vi "FRC-Traj-Lib-SlewRateLimiter-Sample-2.vi"() -> ()   [LabVIEW 2019]
uses:
  <vilib>/Rock Robotics/WPI/ThirdParty/JAS_Junk/TrajLib/Trajectory_Library.lvlib
panel:
  in  "Tab Control":enum32{"Control Panel", "Logic"}(tab)
  in  "Rate Limit  \nMax Units/Sec":dbl=10.0
  in  "Raw Input":dbl(slide)=10.0 scale=-100.0..100.0
  out "Rate Limited Output":dbl
  in  "Enable":bool
  out "Trend":cluster{"Input":dbl, "Output":dbl}(graph)
  out "Rate Limiting Enabled":bool
  # "Slew Rate Limiter Sample 2"
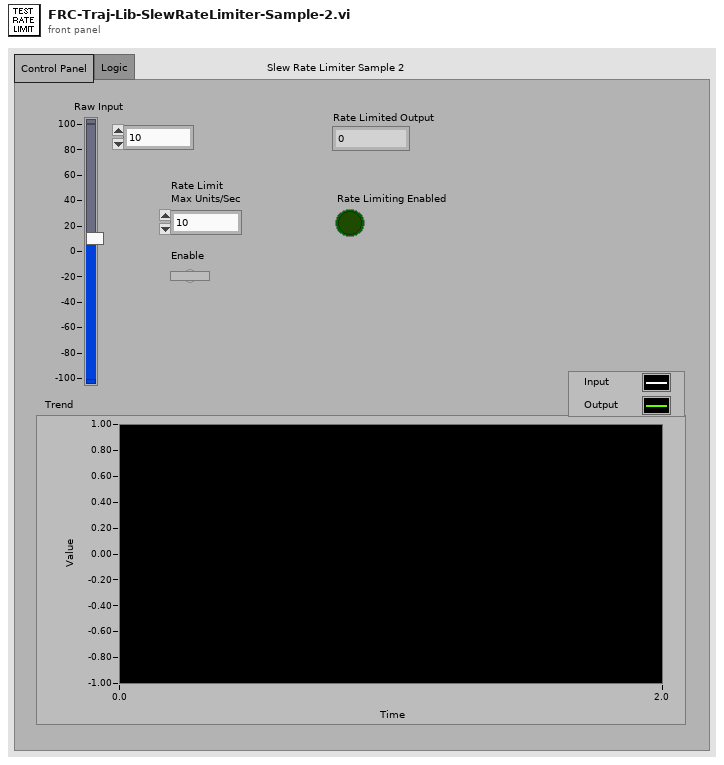
[diagram p1: front panel]
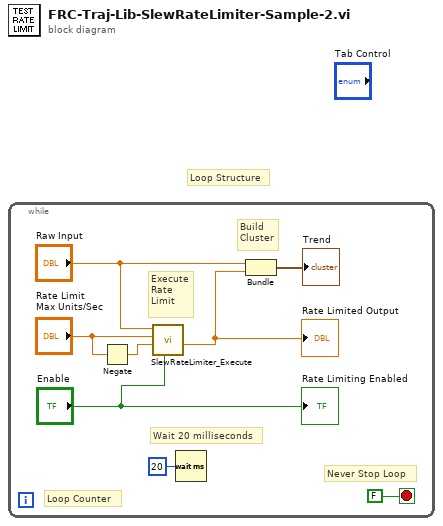
[diagram p0: block diagram]
diagram:
  # "Loop Structure"
  n1 = while {
    stop <- FALSE stop-if-true
    # "Execute\nRate\nLimit"
    # "Build\nCluster"
    # "Loop Counter"
    # "Never Stop Loop"
    # "Wait 20 milliseconds"
    n2 = Negate(x="Rate Limit  \nMax Units/Sec") -> (-x=w1:dbl)
    n3 = call <vilib>:"SlewRateLimiter_Execute.vi"("Enable"="Enable", "NegativeRate"=w1, "PositiveRate"="Rate Limit  \nMax Units/Sec", "Input"="Raw Input") -> ("Output"=w4:dbl)  [unwired: 6 in, 1 out]
    "Rate Limited Output" <- w4
    n4 = Wait (ms)(milliseconds to wait=u32 20) -> ()  [unwired: 1 out]
    n5 = Bundle("Raw Input"="Raw Input", "Output"=w4) -> (→"Trend":cluster{"Raw Input":dbl, "Output":dbl})  [unwired: 1 in]
    "Rate Limiting Enabled" <- "Enable"
  }
